vi "Host - Get ECAT Module Data.vi"(8 "error in (no error)":errorcluster, 11 "ECAT Modules":refnum<k21>[](array[refnum])) -> (0 "error out":errorcluster, 3 "Modules":T1[](array[typedef]))   [LabVIEW 2020, in "SEECD System Explorer.lvlib"]
uses:
  Type Defs/Host - Module.ctl
  Type Defs/IOV Container Contents.ctl
  SEECD System Explorer.lvlib
  <resource>/objmgr/IndComECAT.rc
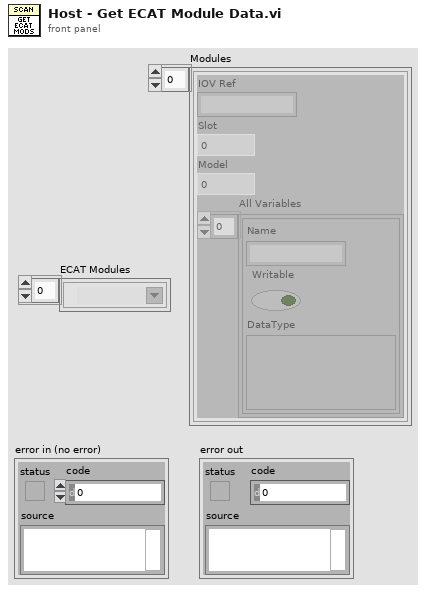
[diagram p1: front panel]
types:
  T1 = typedef "SEECD System Explorer.lvlib/Host - Module.ctl" = cluster{"IOV Ref":string, "Slot":u32, "Model":u32, "All Variables":T2[]}
  T2 = typedef "SEECD System Explorer.lvlib/IOV Container Contents.ctl" = cluster{"Name":string, "Writable":bool, "DataType":variant}
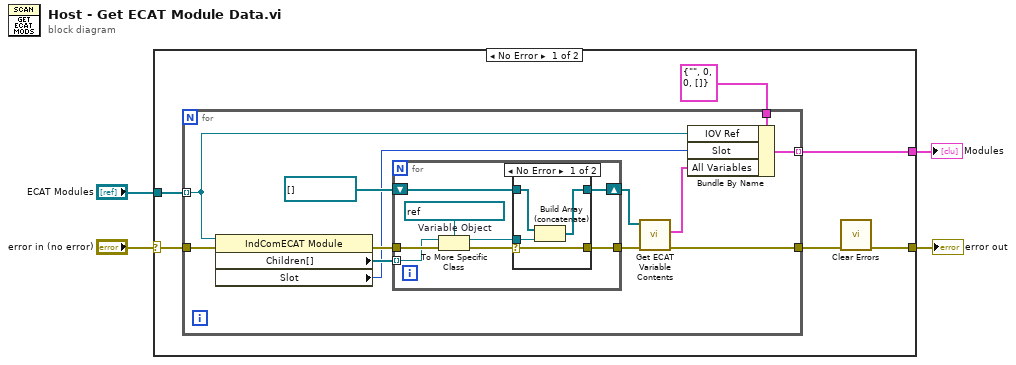
[diagram p0: block diagram]
diagram:
  n1 = case shown="No Error" "error in (no error)" {
    selector: "error in (no error)" -> [w10 w37]
    tunnel: [w7 w37] -> w4
    tunnel: "ECAT Modules" -> [w9 _]
    tunnel: [w5 _] -> w1
    frame No Error {
      n2 = for {
        tunnel: w9 -> [w14] mode=indexing
        tunnel: w10 -> [w22]
        tunnel: [w16] -> w8
        tunnel: T1 {"IOV Ref"="", "Slot"=0, "Model"=0, "All Variables"=[]} ("Module") -> [w15]
        tunnel: [w11] -> w5 mode=indexing
        n3 = property class="IndComECAT Module"(reference=w14, error in=w22) -> (error out=w21:errorcluster, "Children[]"=w19:refnum<k21>[], "Slot"=w13:u32)  [unwired: 1 out]
        n4 = for {
          tunnel: w21 -> [w29]
          tunnel: w19 -> [w25] mode=indexing
          tunnel: [w24] -> w17
          shift-right: [w23] -> w18
          shift-left: refnum<k21>[] [] -> [w27]
          w30 = refnum<k21> refnum  # Variable Object
          n5 = To More Specific Class(target class=w30, reference=w25, error in=w29) -> (specific class reference=w26:refnum<k21>, error out=w28:errorcluster)
          n6 = case shown="No Error" w28 {
            selector: w28 -> [w32 w36]
            tunnel: w27 -> [w34 w35]
            tunnel: w26 -> [w33 _]
            tunnel: [w32 w36] -> w24
            tunnel: [w31 w35] -> w23
            frame No Error {
              n7 = Build Array (concatenate)(w34, w33) -> (w31:refnum<k21>[])
            }
            frame Error {
            }
          }
        }
        n8 = call "Get ECAT Variable Contents.vi"("error in (no error)"=w17, "ECAT Variablenobjekt in"=w18) -> ("error out"=w16:errorcluster, "All Variables Contents"=w12:T2[])  [unwired: 7 in, 1 out]
        n9 = Bundle By Name(cluster=w15, "IOV Ref"=w14, "Slot"=w13, "All Variables"=w12) -> (w11:T1)
      }
      n10 = call <vilib>:"Clear Errors.vi"("error in (no error)"=w8) -> ("error out"=w7:errorcluster)  [unwired: 5 in, 1 out]
    }
    frame Error {
    }
  }
  "Modules" <- w1
  "error out" <- w4
